vi "1_1_matrix_matrix_multiply.vi"(1 "p":i32, 3 "n":i32, 4 "m":i32, 5 "B":fxp<+/-,32,16>[](array[numeric]), 6 "A":fxp<+/-,32,16>[](array[numeric])) -> (0 "C":fxp<+/-,32,16>[](array[numeric]))   [LabVIEW 2020]
panel:
  in  "accum":fxp<+/-,32,16>
  in  "C_type":fxp<+/-,32,16>
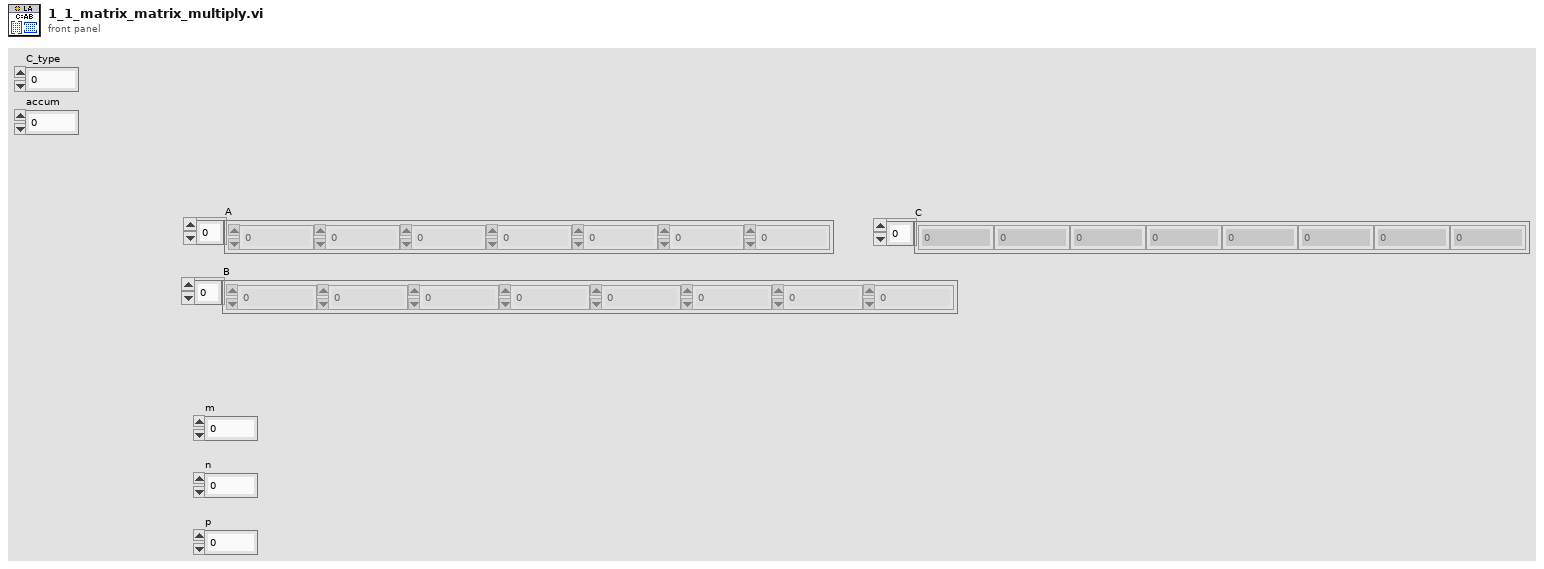
[diagram p1: front panel]
types:
  T1 = enum32{"Extended Precision", "Double Precision", "Single Precision", "Long", "Word", "Byte", "Unsigned Long", "Unsigned Word", "Unsigned Byte", "Complex Extended", "Complex Double", "Complex Single", "Quad", "Unsigned Quad", "Fixed-Point"}
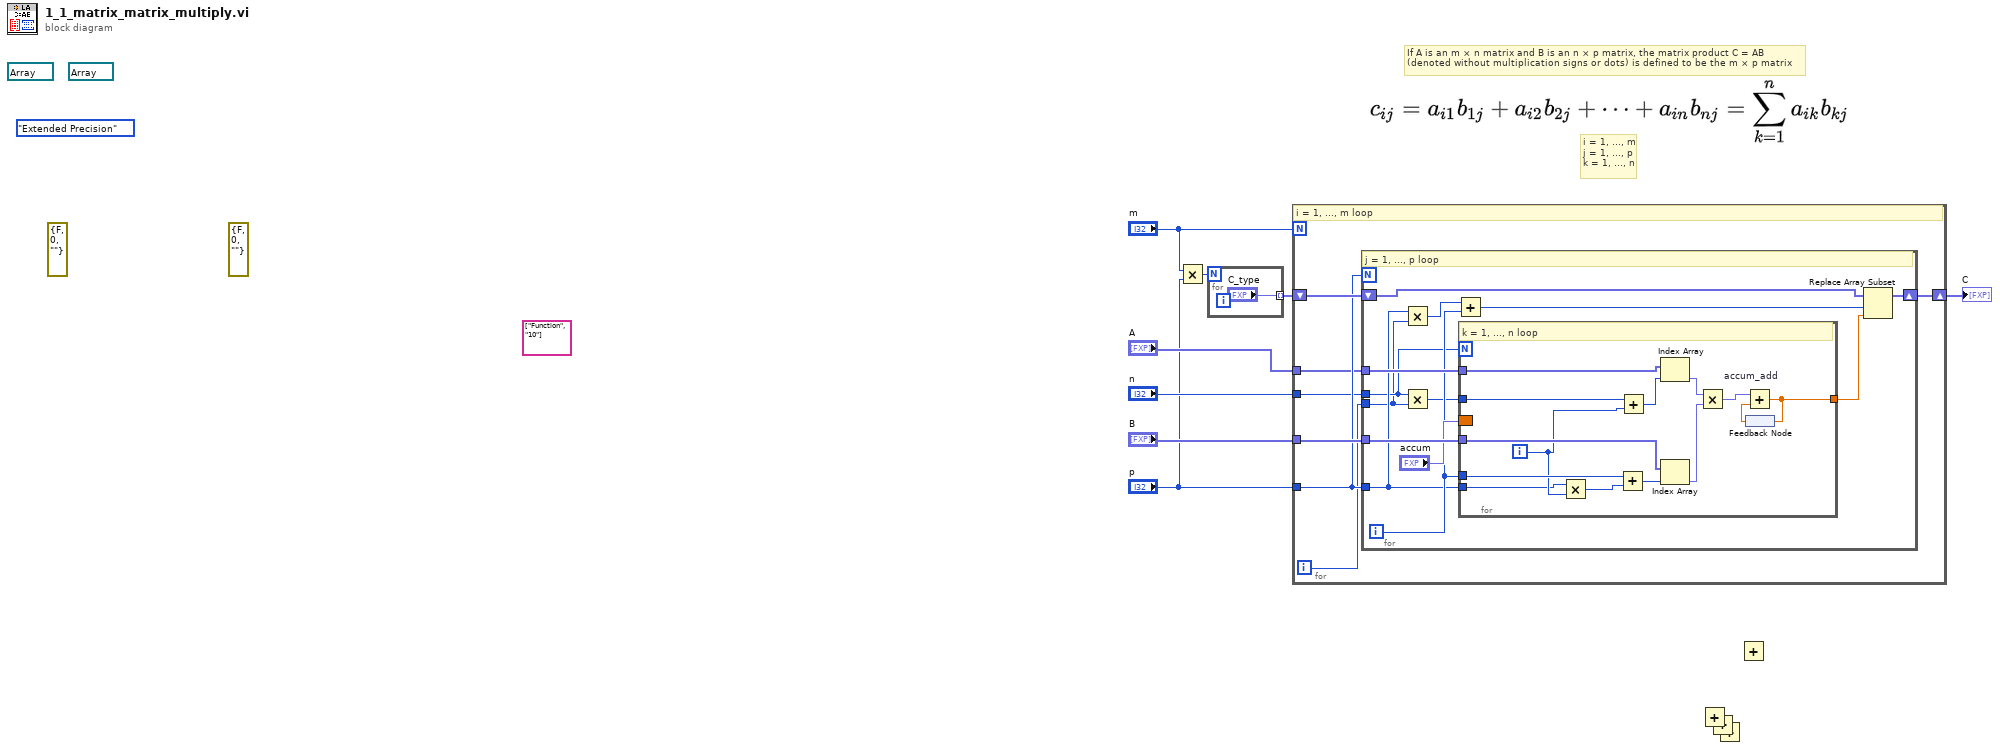
[diagram p0: block diagram]
diagram:
  (unwired) string[][] [["Function", "10"]] ("Traverse All")
  (unwired) refnum<vi> refnum ("Array Ref.")
  (unwired) T1."Extended Precision" ("Representation")
  (unwired) errorcluster {"status"=FALSE, "code"=0, "source"=""} ("error in (no error)")
  (unwired) refnum<vi> refnum ("Ref. Out")
  (unwired) errorcluster {"status"=FALSE, "code"=0, "source"=""} ("error out")
  # "If A is an m × n matrix and B is an n × p matrix, the matrix product C = AB \n(denoted without multiplication signs or dots) is defined to be the m × p matrix"
  # "i = 1, ..., m\nj = 1, ..., p\nk = 1, ..., n"
  n1 = Multiply(x="m", y="p") -> (x*y=w4:i32)
  n2 = for {
    N: w4 -> [_]
    tunnel: ["C_type"] -> w1 mode=indexing
  }
  n3 = for {
    N: "m" -> [_]
    tunnel: "B" -> [w16]
    tunnel: "p" -> [w13]
    tunnel: "A" -> [w12]
    tunnel: "n" -> [w11]
    shift-right: [w14] -> w6
    shift-left: w1 -> [w15]
    i -> [w10]
    # "i = 1, ..., m loop"
    n4 = for {
      N: w13 -> [_]
      tunnel: w12 -> [w29]
      tunnel: w16 -> [w28]
      tunnel: w13 -> [w19]
      shift-right: [w25] -> w14
      shift-left: w15 -> [w26]
      tunnel: w11 -> [w18]
      tunnel: w10 -> [w17]
      i -> [w22]
      # "j = 1, ..., p loop"
      n5 = Multiply(x=w19, y=w17) -> (x*y=w21:i32)
      n6 = Multiply(x=w18, y=w17) -> (x*y=w20:i32)
      n7 = Add(x=w21, y=w22) -> (x+y=w23:i32)
      n8 = for {
        N: w18 -> [_]
        tunnel: w29 -> [w43]
        tunnel: w20 -> [w31]
        tunnel: w28 -> [w42]
        tunnel: w22 -> [w37]
        tunnel: [w30] -> w24
        tunnel: w19 -> [w35]
        border: "accum" -> [_]
        i -> [w36]
        # "k = 1, ..., n loop"
        n9 = Multiply(x=w35, y=w36) -> (x*y=w34:i32)
        n10 = Add(x=w37, y=w34) -> (x+y=w33:i32)
        n11 = Add(x=w31, y=w36) -> (x+y=w32:i32)
        n12 = Index Array(array=w43, index=w32) -> (element=w41:fxp<+/-,32,16>)
        n13 = Index Array(array=w42, index=w33) -> (element=w40:fxp<+/-,32,16>)
        n14 = Multiply(x=w41, y=w40) -> (x*y=w39:fxp<+/-,64,32>)
        n15 = feedback #1() -> (w38:dbl)
        n16 = Add "accum_add"(x=w39, y=w38) -> (x+y=w30:dbl)
        n17 = feedback-in #1(w30) -> ()
      }
      n18 = Replace Array Subset(array=w26, new element=w24, index=w23) -> (w25:fxp<+/-,32,16>[])
    }
  }
  "C" <- w6
  n19 = Add() -> ()  [unwired: 2 in, 1 out]
  n20 = Add() -> ()  [unwired: 2 in, 1 out]
  n21 = Add() -> ()  [unwired: 2 in, 1 out]
  n22 = Add() -> ()  [unwired: 2 in, 1 out]
